vi "Dipper Fridge Resistance Measurement 1.7.vi"() -> ()   [LabVIEW 2011]
panel:
  out "Current Resistance":string
  in  "error in (no error) 3":errorcluster
  out "Sample Cell":string
  in  "error in (no error)":errorcluster
  in  "Heater option":string
  out "3He pot":string
  in  "Lakeshore":bool
  out "Sample Vs. Temp":cluster{dbl[], dbl[]}(graph)
  out "Warning":string="Can't be smaller than 1 s"
  in  "Time delay":u32
  in  "Timer":bool caption="Reset"
  out "Time Elapsed":string
  in  "Save":bool
  out "var":i32
  in  "error in (no error) 2":errorcluster
  out "Heater":bool
  in  "Heater":bool
  out "Boolean":bool
  in  "Power":bool
  in  "Date format (0)":enum16{"short", "long", "abbreviated"}(ring)
  out "size (in bytes)":i64
  out "Calibration":cluster{dbl[], dbl[]}(graph)
  in  "File Path":path
  out "current time":timestamp
  out "Number of Data points":i32
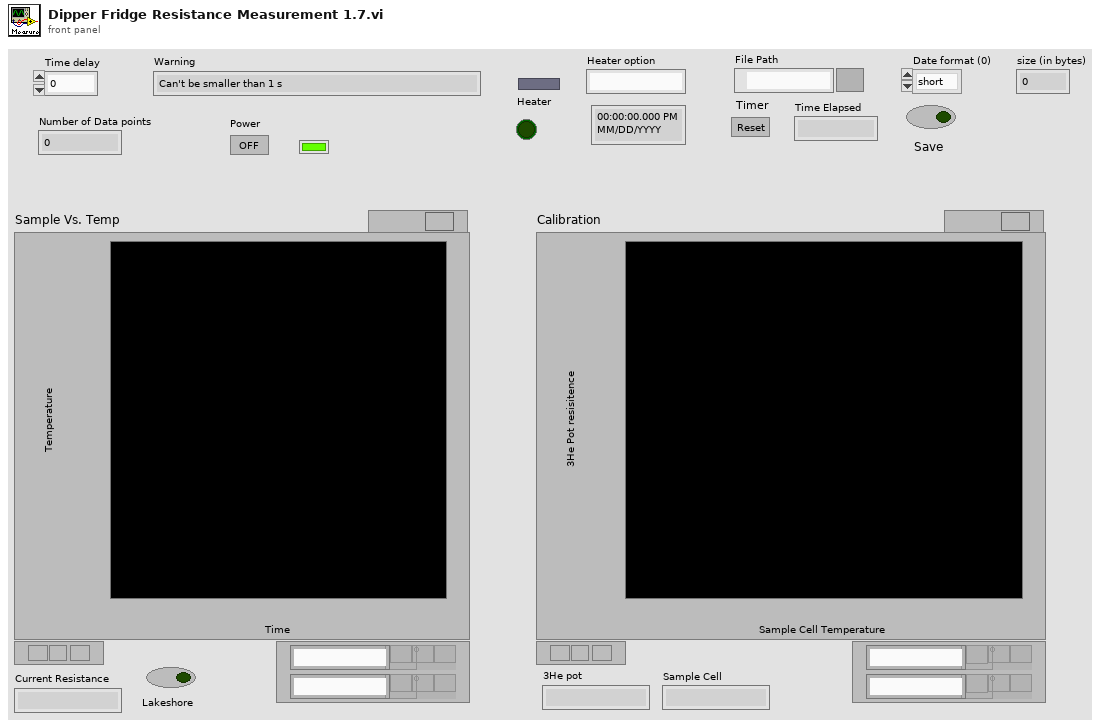
[diagram p1: front panel]
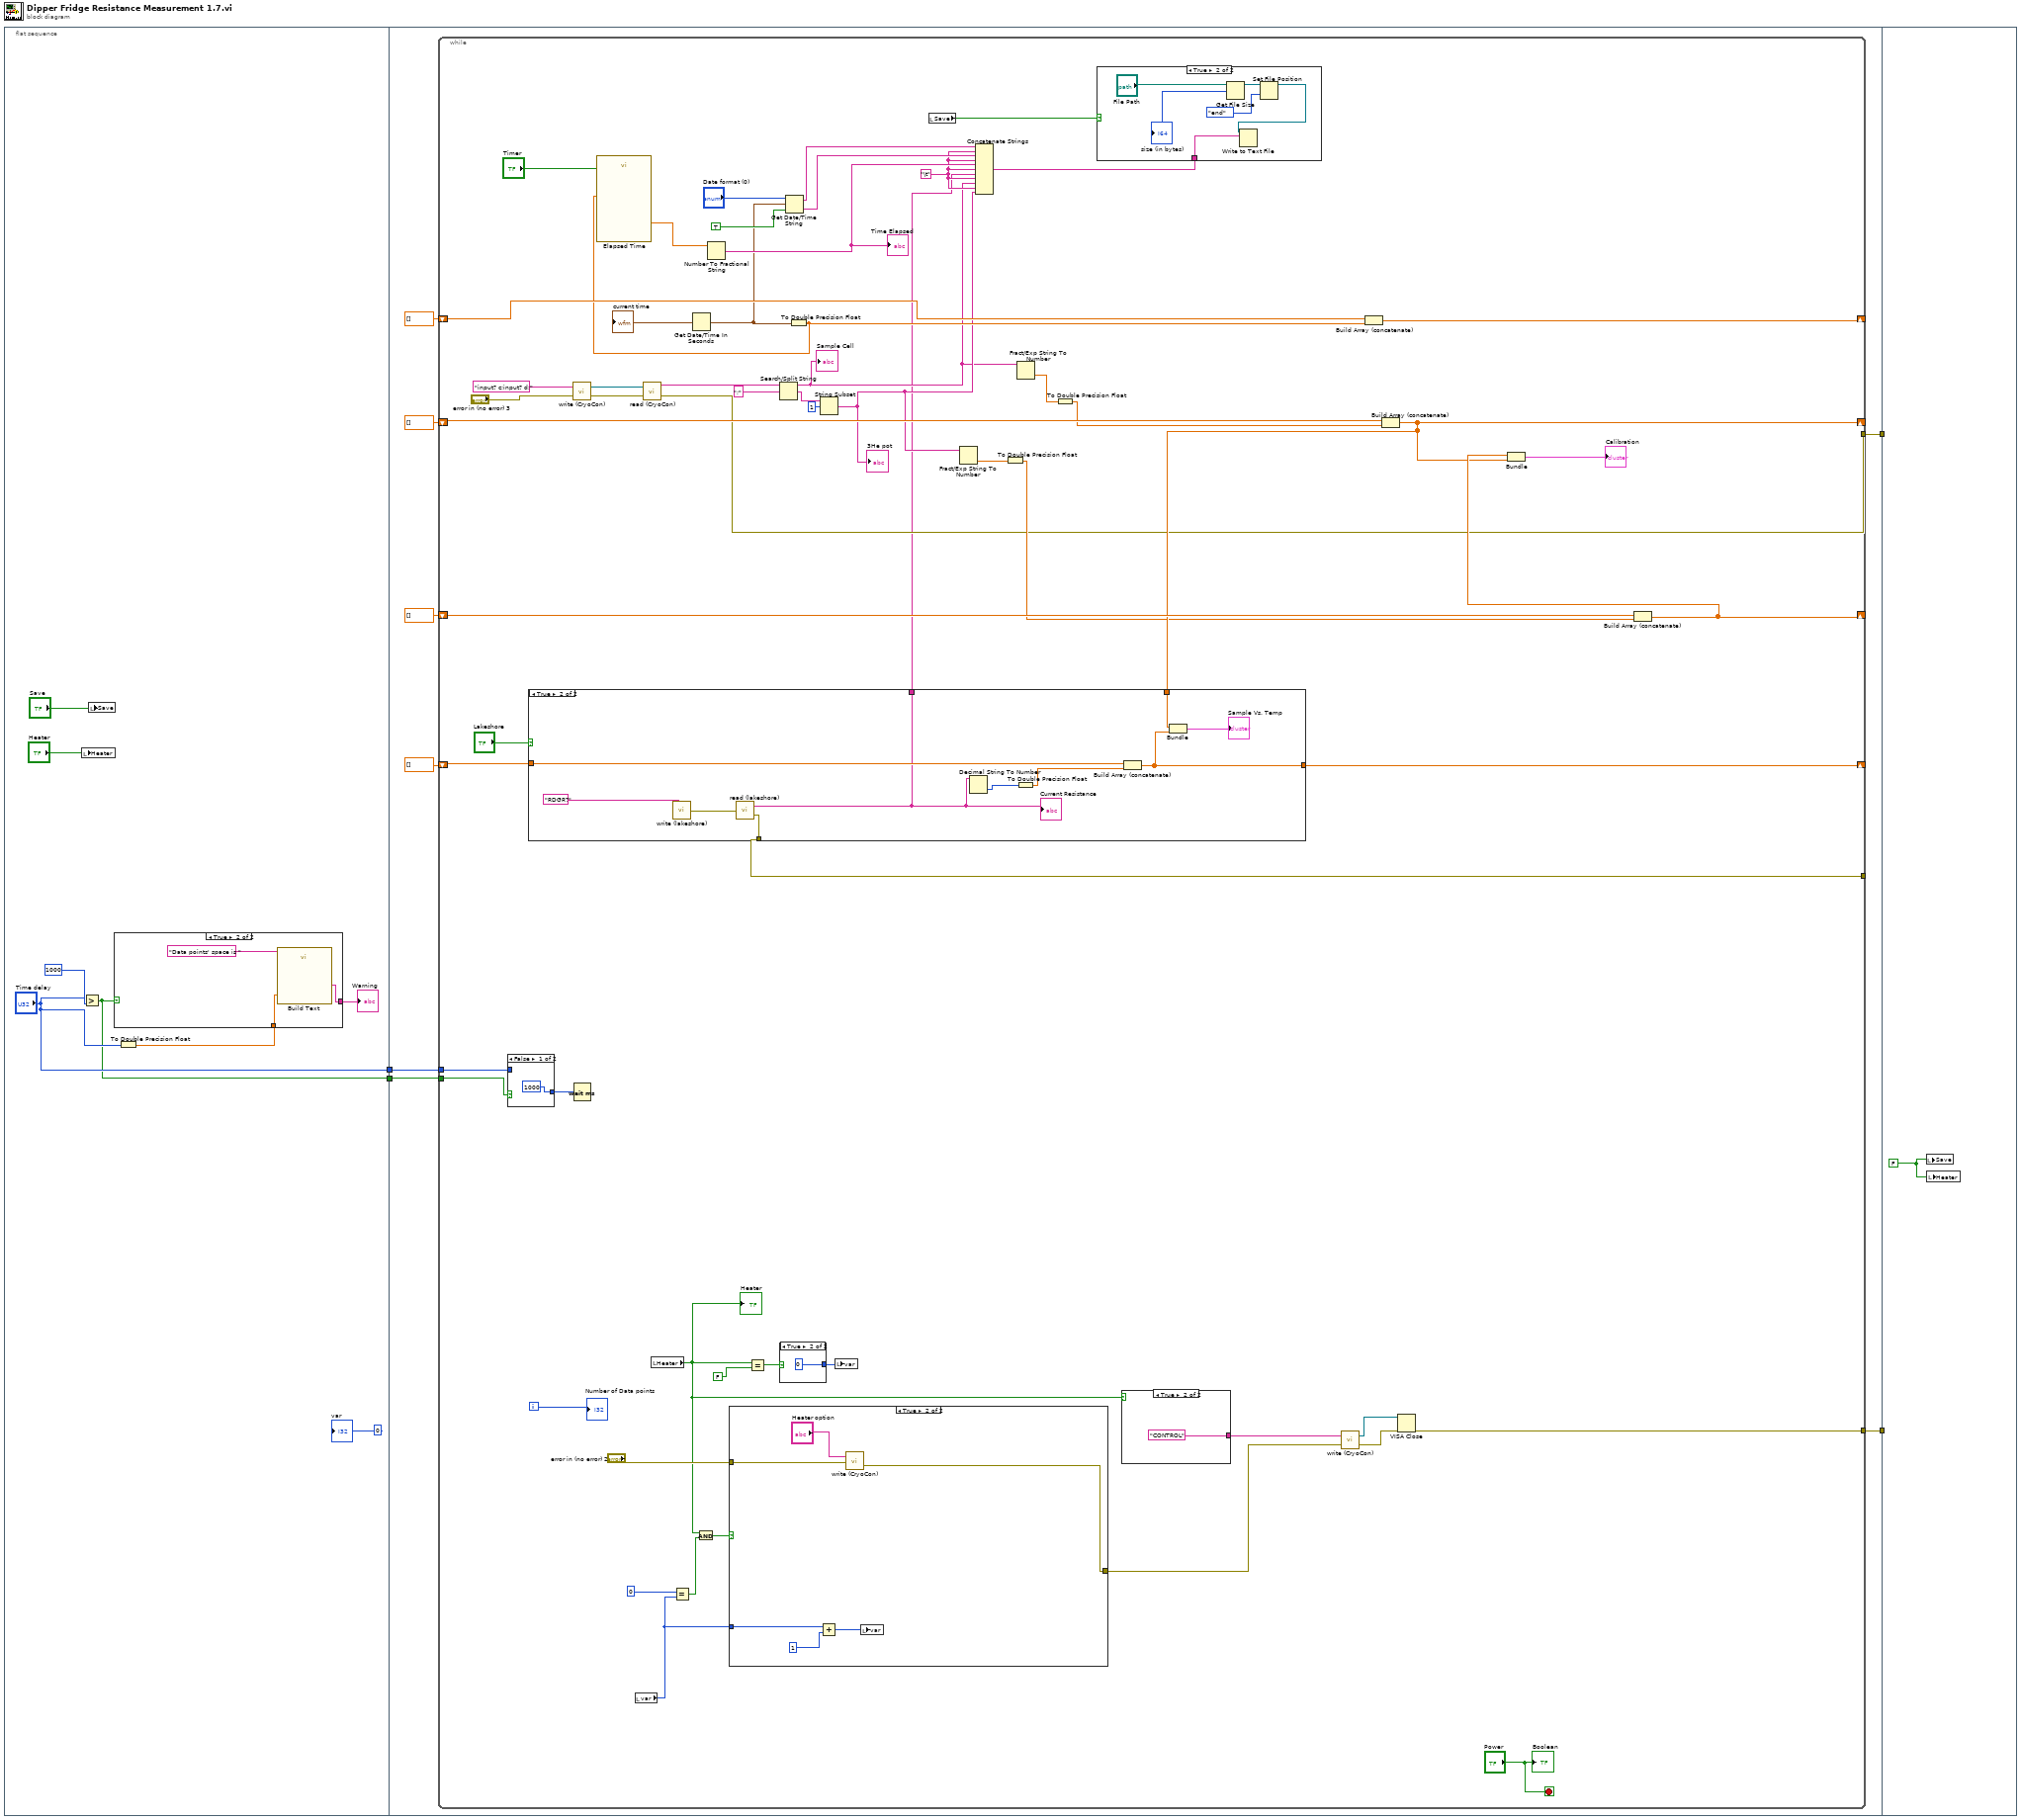
[diagram p0: block diagram]
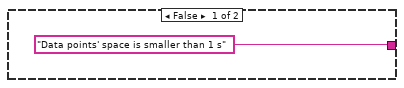
[diagram p2: hidden frame]
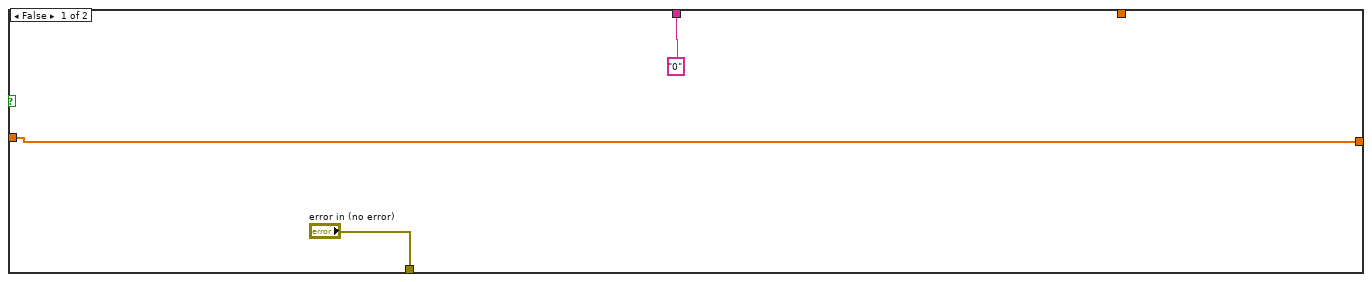
[diagram p3: hidden frame]
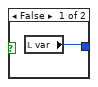
[diagram p5: hidden frame]
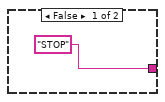
[diagram p7: hidden frame]
diagram:
  n1 = flat-sequence {
    tunnel: ["Time delay"] -> w4
    tunnel: [w5] -> w3
    tunnel: w4 -> [w20]
    tunnel: w3 -> [w19]
    tunnel: [w18] -> w2
    tunnel: [w17] -> w1
    tunnel: w2 -> [_]
    tunnel: w1 -> [_]
    frame #0 {
      n2 = local write "Heater"("Heater") -> ()
      n3 = Greater?(x="Time delay", y=u32 1000 ("x")) -> (0:w5:bool)
      n4 = local write "Save"("Save") -> ()
      n5 = To Double Precision Float(number="Time delay") -> (double precision float=w7:dbl)
      n6 = case shown="True" w5 {
        tunnel: w7 -> [_ w14]
        tunnel: ["Data points' space is smaller than 1 s" w16] -> w8
        frame False {
        }
        frame True {
          n7 = call "Build Text"("Beginning Text"="Data points' space is ", "Y"=w14) -> ("Result"=w16:string)  [unwired: 12 in, 1 out]
        }
      }
      "Warning" <- w8
      "var" <- 0 ("var")
    }
    frame #1 {
      n8 = while {
        tunnel: [w81] -> _
        shift-right: [w48] -> _
        shift-left: dbl[] [] -> [w78]
        shift-right: [w41] -> _
        shift-left: dbl[] [] -> [w75]
        shift-right: [w46] -> _
        shift-left: dbl[] [] -> [w53]
        shift-right: [w42] -> _
        shift-left: dbl[] [] -> [w52]
        tunnel: w20 -> [w49]
        tunnel: w19 -> [w50]
        tunnel: [w33] -> w18
        tunnel: [w28] -> w17
        i -> [w80]
        stop <- "Power" stop-if-true
        w47 = "\t"
        n9 = case shown="False" w50 {
          tunnel: [1000 w97] -> w51
          tunnel: w49 -> [_ w97]
          frame False {
          }
          frame True {
          }
        }
        n10 = call "write (CryoCon).vi"("error in (no error)"="error in (no error) 3", "write buffer"="input? c;input? d;") -> ("error out"=w31:errorcluster, "VISA resource name out"=w32:refnum<visa-resource-name>)
        n11 = Wait (ms)(milliseconds to wait=w51) -> ()  [unwired: 1 out]
        n12 = local read "var"() -> (w70:i32)
        n13 = call "read (CryoCon).vi"("error in (no error)"=w31, "VISA resource name"=w32) -> ("error out"=w33:errorcluster, "read buffer"=w34:string)
        n14 = local read "Heater"() -> (w61:bool)
        "Heater" <- w61
        n15 = Equal?(x=0, y=w70) -> (x = y?=w68:bool)
        n16 = Get Date/Time In Seconds() -> (seconds since 1Jan1904=w59:timestamp)
        "current time" <- w59
        n17 = And(x=w61, y=w68) -> (x .and. y?=w67:bool)
        n18 = case shown="True" w67 {
          tunnel: [w100 w101] -> w66
          tunnel: "error in (no error) 2" -> [w100 w103]
          tunnel: w70 -> [_ w106]
          frame False {
          }
          frame True {
            n19 = Add(x=w106, y=1) -> (x+y=w104:i32)
            n20 = call "write (CryoCon).vi"("error in (no error)"=w103, "write buffer"="Heater option") -> ("error out"=w101:errorcluster)  [unwired: 1 out]
            n21 = local write "var"(w104) -> ()
          }
        }
        n22 = Equal?(x=w61, y=FALSE ("Heater")) -> (x = y?=w63:bool)
        n23 = Search/Split String(string=w34, search string/char (-)=";") -> (substring before match=w26:string, match + rest of string=w37:string)  [unwired: 1 in, 1 out]
        "Sample Cell" <- w26
        n24 = case shown="True" w63 {
          tunnel: [w98 0] -> w62
          frame False {
            n25 = local read "var"() -> (w98:i32)
          }
          frame True {
          }
        }
        n26 = Get Date/Time String(date format (0)="Date format (0)", seconds (now)=w59, want seconds? (F)=TRUE) -> (date string=w54:string, time string=w55:string)
        n27 = To Double Precision Float(number=w59) -> (double precision float=w57:dbl)
        n28 = call "Elapsed Time"("Reset"="Timer", "Set Start Time (s)"=w57) -> ("Elapsed Time (s)"=w58:dbl)  [unwired: 10 in, 7 out]
        n29 = Number To Fractional String(number=w58) -> (F-format string=w60:string)  [unwired: 3 in]
        "Time Elapsed" <- w60
        n30 = String Subset(string=w37, offset (0)=1) -> (substring=w27:string)  [unwired: 1 in]
        "3He pot" <- w27
        n31 = local write "var"(w62) -> ()
        n32 = local read "Save"() -> (w65:bool)
        n33 = Fract/Exp String To Number(string=w27) -> (number=w39:dbl)  [unwired: 3 in, 1 out]
        n34 = To Double Precision Float(number=w39) -> (double precision float=w38:dbl)
        n35 = Fract/Exp String To Number(string=w26) -> (number=w45:dbl)  [unwired: 3 in, 1 out]
        n36 = To Double Precision Float(number=w45) -> (double precision float=w44:dbl)
        n37 = case shown="True" w61 {
          tunnel: ["STOP" ("write buffer") "CONTROL" ("write buffer")] -> w72
          frame False {
          }
          frame True {
          }
        }
        n38 = call "write (CryoCon).vi"("error in (no error)"=w66, "write buffer"=w72) -> ("error out"=w29:errorcluster, "VISA resource name out"=w30:refnum<visa-resource-name>)
        n39 = Build Array (concatenate)(w78, w57) -> (w48:dbl[])
        n40 = Build Array (concatenate)(w75, w44) -> (w41:dbl[])
        n41 = case shown="True" "Lakeshore" {
          tunnel: ["error in (no error)" w95] -> w81
          tunnel: w53 -> [w84 w92]
          tunnel: ["0" ("read buffer") w91] -> w25
          tunnel: [w84 w88] -> w46
          tunnel: w41 -> [_ w86]
          frame False {
          }
          frame True {
            n42 = call "write (lakeshore).vi"("write buffer"="RDGR?") -> ("error out"=w94:errorcluster)  [unwired: 1 in]
            n43 = call "read (lakeshore).vi"("error in (no error)"=w94) -> ("read buffer"=w91:string, "error out"=w95:errorcluster)
            "Current Resistance" <- w91
            n44 = Decimal String To Number(string=w91) -> (number=w90:i32)  [unwired: 2 in, 1 out]
            n45 = To Double Precision Float(number=w90) -> (double precision float=w89:dbl)
            n46 = Build Array (concatenate)(w92, w89) -> (w88:dbl[])
            n47 = Bundle(w86, w88) -> (→"Sample Vs. Temp":cluster{dbl[], dbl[]})  [unwired: 1 in]
          }
        }
        n48 = Concatenate Strings(w54, w47, w55, w47, w60, w47, w25, w47, w26, w47, w27) -> (w77:string)
        n49 = case shown="True" w65 {
          tunnel: w77 -> [_ w114]
          frame False {
          }
          frame True {
            n50 = Get File Size(file="File Path") -> (refnum out=w112:refnum<file>, size (in bytes)=→"size (in bytes)":i64)  [unwired: 1 in, 1 out]
            n51 = Set File Position(refnum=w112, from (0:start)=enum16{"start", "end", "current"}."end") -> (refnum out=w111:refnum<file>)  [unwired: 2 in, 1 out]
            n52 = Write to Text File(file (use dialog)=w111, text=w114) -> ()  [unwired: 2 in, 3 out]
          }
        }
        n53 = VISA Close(VISA resource name=w30, error in (no error)=w29) -> (error out=w28:errorcluster)
        n54 = Build Array (concatenate)(w52, w38) -> (w42:dbl[])
        n55 = Bundle(w42, w41) -> (→"Calibration":cluster{dbl[], dbl[]})  [unwired: 1 in]
        "Number of Data points" <- w80
        "Boolean" <- "Power"
      }
    }
    frame #2 {
      w115 = FALSE ("Save")
      n56 = local write "Save"(w115) -> ()
      n57 = local write "Heater"(w115) -> ()
    }
  }
